vi "CheckLocation.vi"(0 "Message Queue":refnum<queue>, 1 "Waypoint Array Size":i32, 5 "Waypoint Array (in)":cluster{"Latitude":dbl, "Longitude":dbl}[](array[cluster]), 9 "GPS Data":T1, 11 "error (in)":errorcluster) -> (6 "Waypoint Array (out)":cluster{"Latitude":dbl, "Longitude":dbl}[](array[cluster]), 12 "En Route":i32, 13 "Waypoints remaining":i32, 14 "Progress Bar":u8(slide) scale=0.0..100.0, 15 "error (out)":errorcluster)   [LabVIEW 2015]
doc: "Checks to see if the waypoint has been reached. If it has then the next waypoint in the array is selected as the current destination. Special case for the last waypoint (return home). Deceleration sequence is then initiated."
uses:
  support/Message Queue/Message Cluster.ctl
  support/Message Queue/Enqueue Message (Single).vi
  support/Message Queue/Message Queue.lvlib
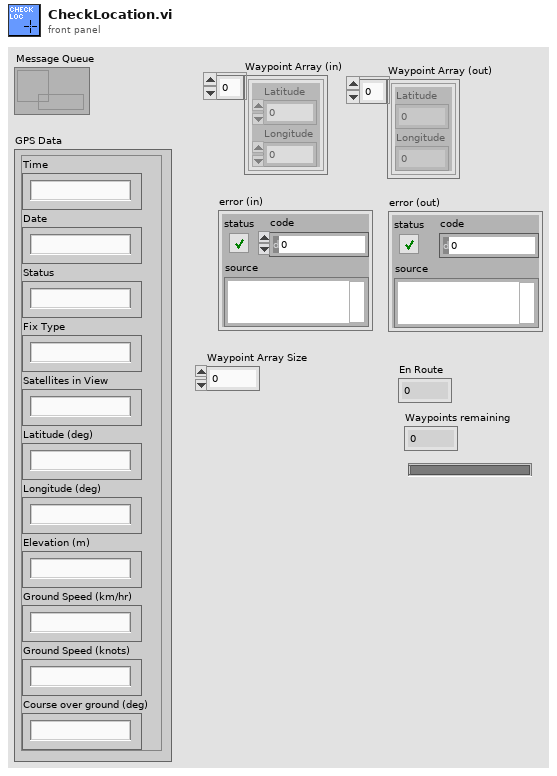
[diagram p1: front panel]
types:
  T1 = cluster{"Time":string, "Date":string, "Status":string, "Fix Type":string, "Satellites in View":string, "Latitude (deg)":string, "Longitude (deg)":string, "Elevation (m)":string, "Ground Speed (km/hr)":string, "Ground Speed (knots)":string, "Course over ground (deg)":string}
  T2 = enum16{"Current Destination", "Next Destination"}
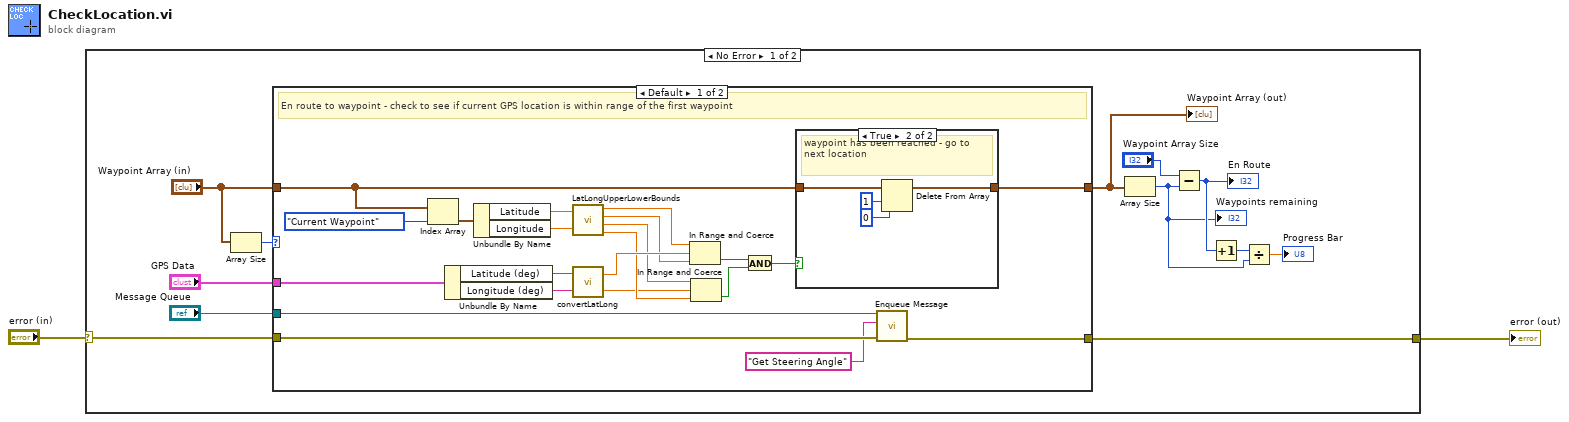
[diagram p0: block diagram]
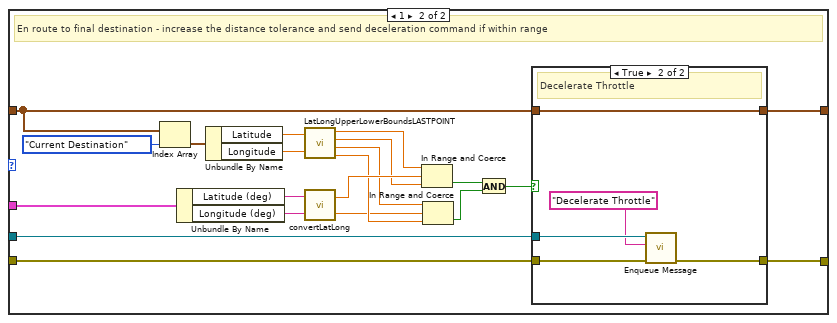
[diagram p3: hidden frame]
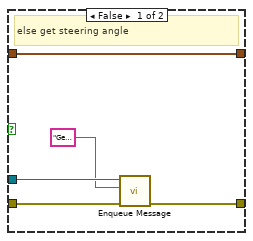
[diagram p4: hidden frame]
diagram:
  n1 = case shown="No Error" "error (in)" {
    selector: "error (in)" -> [w13 w73]
    tunnel: [w9 w73] -> w1
    frame No Error {
      n2 = Array Size(array="Waypoint Array (in)") -> (size(s)=w14:i32)
      n3 = case shown="Default" w14 {
        tunnel: w13 -> [w17 w46]
        tunnel: "GPS Data" -> [w34 w50]
        tunnel: "Waypoint Array (in)" -> [w20 w44]
        tunnel: [w19 w43] -> w8
        tunnel: "Message Queue" -> [w18 w45]
        tunnel: [w15 w42] -> w9
        frame Default {
          # "En route to waypoint - check to see if current GPS location is within range of the first waypoint"
          n4 = Index Array(array=w20, index=enum16{"Current Waypoint", "Next Destination"}."Current Waypoint") -> (element=w35:cluster{"Latitude":dbl, "Longitude":dbl})
          n5 = Unbundle By Name(w34) -> ("Latitude (deg)"=w33:string, "Longitude (deg)"=w32:string)
          n6 = Unbundle By Name(w35) -> ("Latitude"=w30:dbl, "Longitude"=w29:dbl)
          n7 = call "LatLongUpperLowerBounds.vi"("Latitude"=w30, "Longitude"=w29) -> ("Lat Upper"=w28:dbl, "Lat Lower"=w27:dbl, "Long Upper"=w26:dbl, "Long Lower"=w25:dbl)
          n8 = call "convertLatLong.vi"("Longitude (deg)"=w32, "Latitude (deg)"=w33) -> ("Longitude (deg)"=w24:dbl, "Latitude (deg)"=w31:dbl)
          n9 = In Range and Coerce(upper limit=w28, x=w31, lower limit=w27) -> (In Range?=w23:bool)  [unwired: 1 out]
          n10 = In Range and Coerce(upper limit=w26, x=w24, lower limit=w25) -> (In Range?=w22:bool)  [unwired: 1 out]
          n11 = And(x=w23, y=w22) -> (x .and. y?=w21:bool)
          n12 = case shown="True" w21 {
            tunnel: w20 -> [w37 w41]
            tunnel: [w37 w38] -> w19
            frame False {
              # "waypoint has not been reached - continue to current waypoint"
            }
            frame True {
              # "waypoint has been reached - go to next location"
              n13 = Delete From Array(array=w41, length=1, index=0) -> (array with subset deleted=w38:cluster{"Latitude":dbl, "Longitude":dbl}[])  [unwired: 1 out]
            }
          }
          n14 = call-poly "Enqueue Message.vi"("error in (no error)"=w17, "Message"="Get Steering Angle", "Message Queue"=w18) -> ("error out"=w15:errorcluster)  [unwired: 7 in, 1 out]
        }
        frame 1 {
          # "En route to final destination - increase the distance tolerance and send deceleration command if within range"
          n15 = Index Array(array=w44, index=T2."Current Destination") -> (element=w61:cluster{"Latitude":dbl, "Longitude":dbl})
          n16 = Unbundle By Name(w50) -> ("Latitude (deg)"=w60:string, "Longitude (deg)"=w59:string)
          n17 = Unbundle By Name(w61) -> ("Latitude"=w57:dbl, "Longitude"=w56:dbl)
          n18 = call "LatLongUpperLowerBoundsLASTPOINT.vi"("Latitude"=w57, "Longitude"=w56) -> ("Lat Upper"=w55:dbl, "Lat Lower"=w54:dbl, "Long Upper"=w53:dbl, "Long Lower"=w52:dbl)
          n19 = call "convertLatLong.vi"("Longitude (deg)"=w59, "Latitude (deg)"=w60) -> ("Longitude (deg)"=w51:dbl, "Latitude (deg)"=w58:dbl)
          n20 = In Range and Coerce(upper limit=w55, x=w58, lower limit=w54) -> (In Range?=w49:bool)  [unwired: 1 out]
          n21 = In Range and Coerce(upper limit=w53, x=w51, lower limit=w52) -> (In Range?=w48:bool)  [unwired: 1 out]
          n22 = And(x=w49, y=w48) -> (x .and. y?=w47:bool)
          n23 = case shown="True" w47 {
            tunnel: w46 -> [w65 w72]
            tunnel: w45 -> [w66 w71]
            tunnel: w44 -> [w67 w68]
            tunnel: [w67 w68] -> w43
            tunnel: [w63 w70] -> w42
            frame False {
              # "else get steering angle"
              n24 = call-poly "Enqueue Message.vi"("error in (no error)"=w65, "Message"="Get Steering Angle", "Message Queue"=w66) -> ("error out"=w63:errorcluster)  [unwired: 7 in, 1 out]
            }
            frame True {
              # "Decelerate Throttle"
              n25 = call-poly "Enqueue Message.vi"("error in (no error)"=w72, "Message"="Decelerate Throttle", "Message Queue"=w71) -> ("error out"=w70:errorcluster)  [unwired: 7 in, 1 out]
            }
          }
        }
      }
      "Waypoint Array (out)" <- w8
      n26 = Array Size(array=w8) -> (size(s)=w4:i32)
      "Waypoints remaining" <- w4
      n27 = Subtract(x="Waypoint Array Size", y=w4) -> (x-y=w6:i32)
      "En Route" <- w6
      n28 = Increment(x=w6) -> (x+1=w5:i32)
      n29 = Divide(x=w5, y=w4) -> (x/y=→"Progress Bar":dbl)
    }
    frame Error {
    }
  }
  "error (out)" <- w1
